vi "Write Modulation.vi"(8 "error in (no error)":errorcluster, 10 "Modulation":enum8{"Sine", "Square"}[](array[ring]), 11 "Set Modulation MSG in":refnum<class "Set Modulation MSG.lvclass">) -> (0 "error out":errorcluster, 3 "Set Modulation MSG out":refnum<class "Set Modulation MSG.lvclass">)   [LabVIEW 2014, in "ePAS Library.lvlib" / "Set Modulation MSG.lvclass"]
uses:
  Set Modulation MSG.lvclass
  Set Modulation MSG.lvclass/Set Modulation MSG.ctl
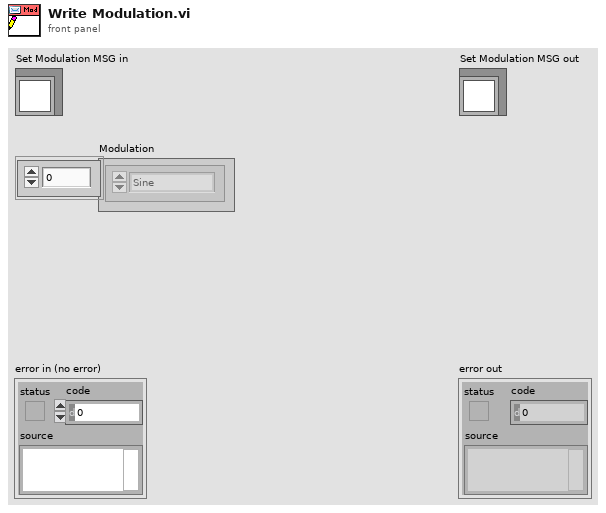
[diagram p1: front panel]
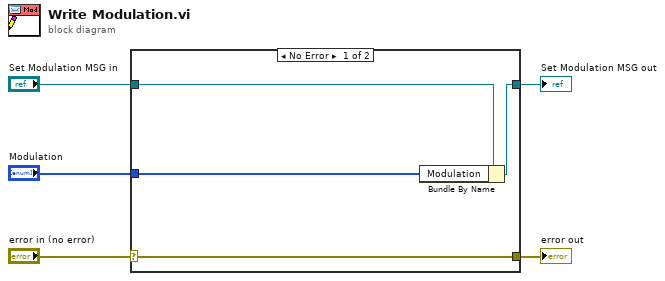
[diagram p0: block diagram]
diagram:
  n1 = case shown="No Error" "error in (no error)" {
    selector: "error in (no error)" -> [w9 w10]
    tunnel: [w9 w10] -> w4
    tunnel: [w7 w11] -> w2
    tunnel: "Set Modulation MSG in" -> [w8 w11]
    tunnel: "Modulation" -> [w6 _]
    frame No Error {
      n2 = Bundle By Name(cluster=w8, "Modulation"=w6) -> (w7:refnum<class "Set Modulation MSG.lvclass">)
    }
    frame Error {
    }
  }
  "error out" <- w4
  "Set Modulation MSG out" <- w2
